vi "LockedState.vi"(8 "error in (no error)":errorcluster, 10 "Player":refnum<class "Player.lvclass">, 11 "LockedState in":refnum<class "LockedState.lvclass">) -> (0 "error out":errorcluster, 3 "LockedState out":refnum<class "LockedState.lvclass">)   [LabVIEW 2018, in "LockedState.lvclass"]
uses:
  LockedState.lvclass
  Player Class/Player.lvclass
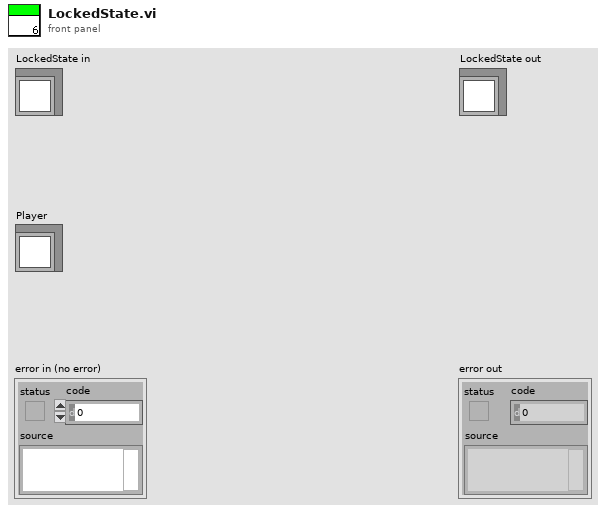
[diagram p1: front panel]
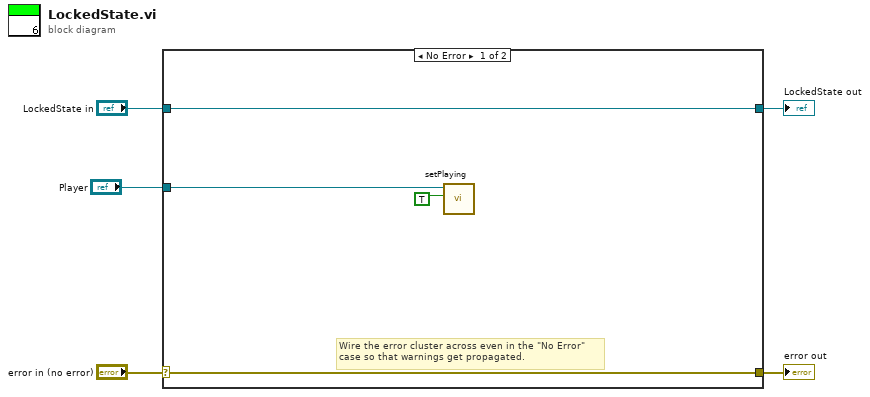
[diagram p0: block diagram]
diagram:
  n1 = case shown="No Error" "error in (no error)" {
    selector: "error in (no error)" -> [w8 w11]
    tunnel: [w8 w11] -> w4
    tunnel: [w9 w10] -> w2
    tunnel: "LockedState in" -> [w9 w10]
    tunnel: "Player" -> [w6 _]
    frame No Error {
      # "Wire the error cluster across even in the \"No Error\"\ncase so that warnings get propagated."
      n2 = call "setPlaying.vi"("playing"=TRUE, "Player in"=w6) -> ()  [unwired: 8 in, 2 out]
    }
    frame Error {
    }
  }
  "error out" <- w4
  "LockedState out" <- w2
